vi "GUI_HTT_1Wire.vi"() -> ()   [LabVIEW 2013]
uses:
  Shared/GUI_Template/GUI_master/tcp_new_data_event.ctl
  Shared/GUI_Template/GUI_master/tcp new data cluster.ctl
panel:
  in  "Position.Channel 10::1":T1(ring) caption="Beamstop South"
  in  "Position.Channel 9::1":T1(ring) caption="Beamstop North"
  in  "Position.Channel 5::1":T1(ring) caption="Amp3 North"
  in  "Position.Channel 8::1":T1(ring) caption="Amp4 South"
  in  "Position.Channel 6::1":T1(ring) caption="Amp3 South"
  in  "Position.Channel 7::1":T1(ring) caption="Amp4 North"
  in  "Position.Channel 4::1":T1(ring) caption="Amp2 South"
  in  "Position.Channel 3::1":T1(ring) caption="Amp2 North"
  in  "Position.Channel 2::1":T1(ring) caption="Revo 1 South"
  in  "Position.Channel 1::1":T1(ring) caption="Revo 1 North"
  out "error IO 2":errorcluster
  out "tcp data event":T2
  in  "UDP error message":string
  in  "GUIdevice 2":string
  in  "GUIdevice 1":string="HTT-1Wire-LCave"
  in  "stop":bool
  # "HTT-1Wire"
  # "Energy"
  # "CAP"
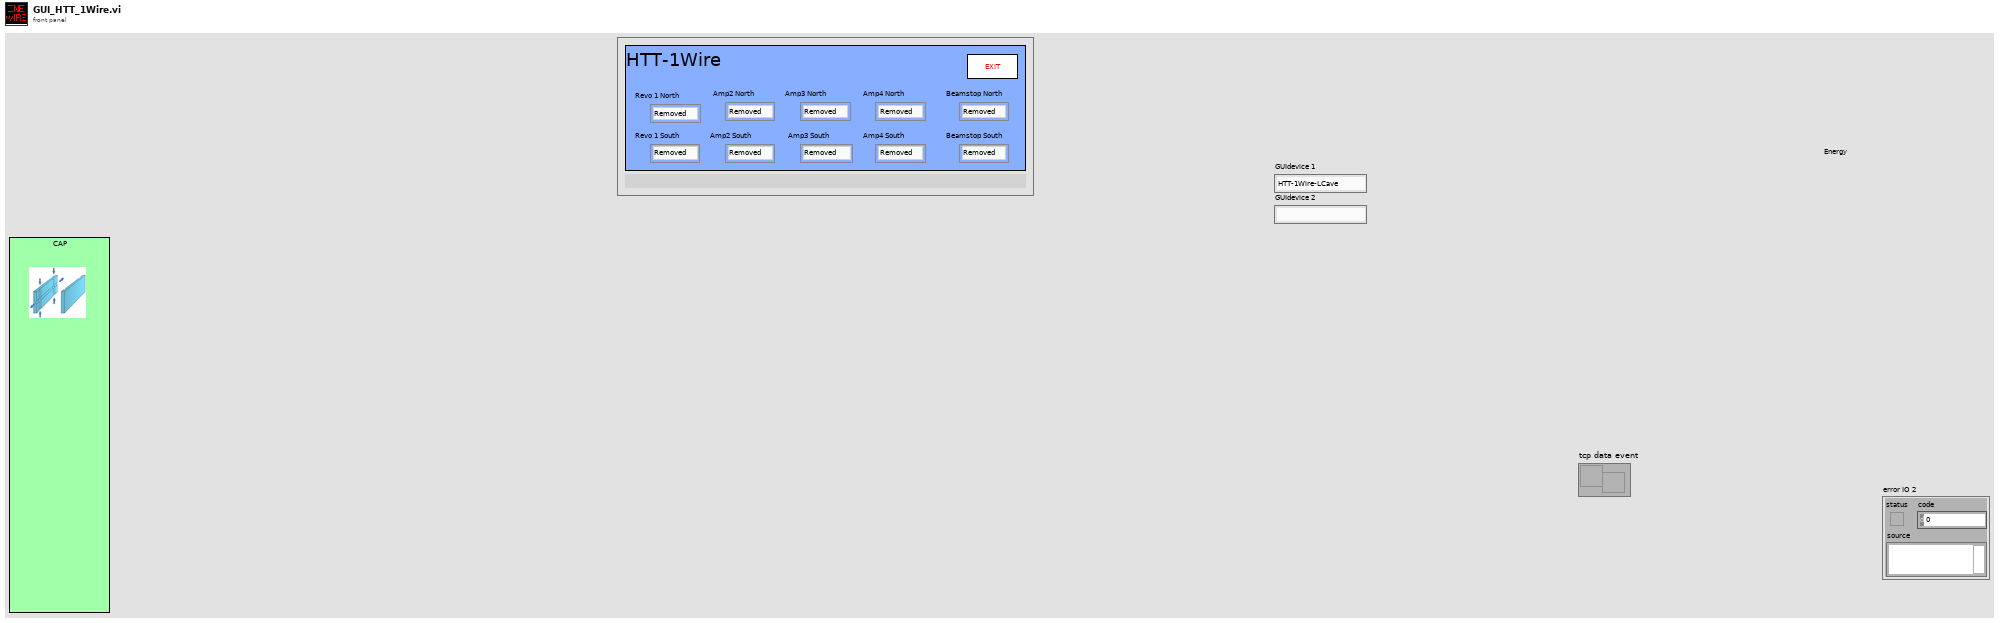
[diagram p1: front panel]
types:
  T1 = enum16{"Removed", "Inserted", "Unknown", "Moving"}
  T2 = typedef "tcp_new_data_event.ctl" = refnum<user-event>
  T3 = typedef "tcp new data cluster.ctl" = cluster{"EventEnum":enum16{"new data", "connection status update"}, "Device name":string}
  T4 = enum32{"invalid app kind", "Development System", "Run Time System", "Student Edition", "Embedded LabVIEW", "Evaluation", "Custom"}
  T5 = enum32{"Invalid", "Standard", "Closed", "Hidden", "Minimized", "Maximized"}
  T6 = cluster{"Core":cluster{"Current VI Reference":refnum<vi>, "Close Panel on Exit?":bool}, "Heater timing offset":dbl, "Discharge timing offset":dbl, "Jet trigger":bool, "Tik1":u32, "Tik2":u32, "Fire Continues Allowed":bool, "Jet enable":bool}
  T7 = cluster{"Current VI Reference":refnum<vi>, "Close Panel on Exit?":bool}
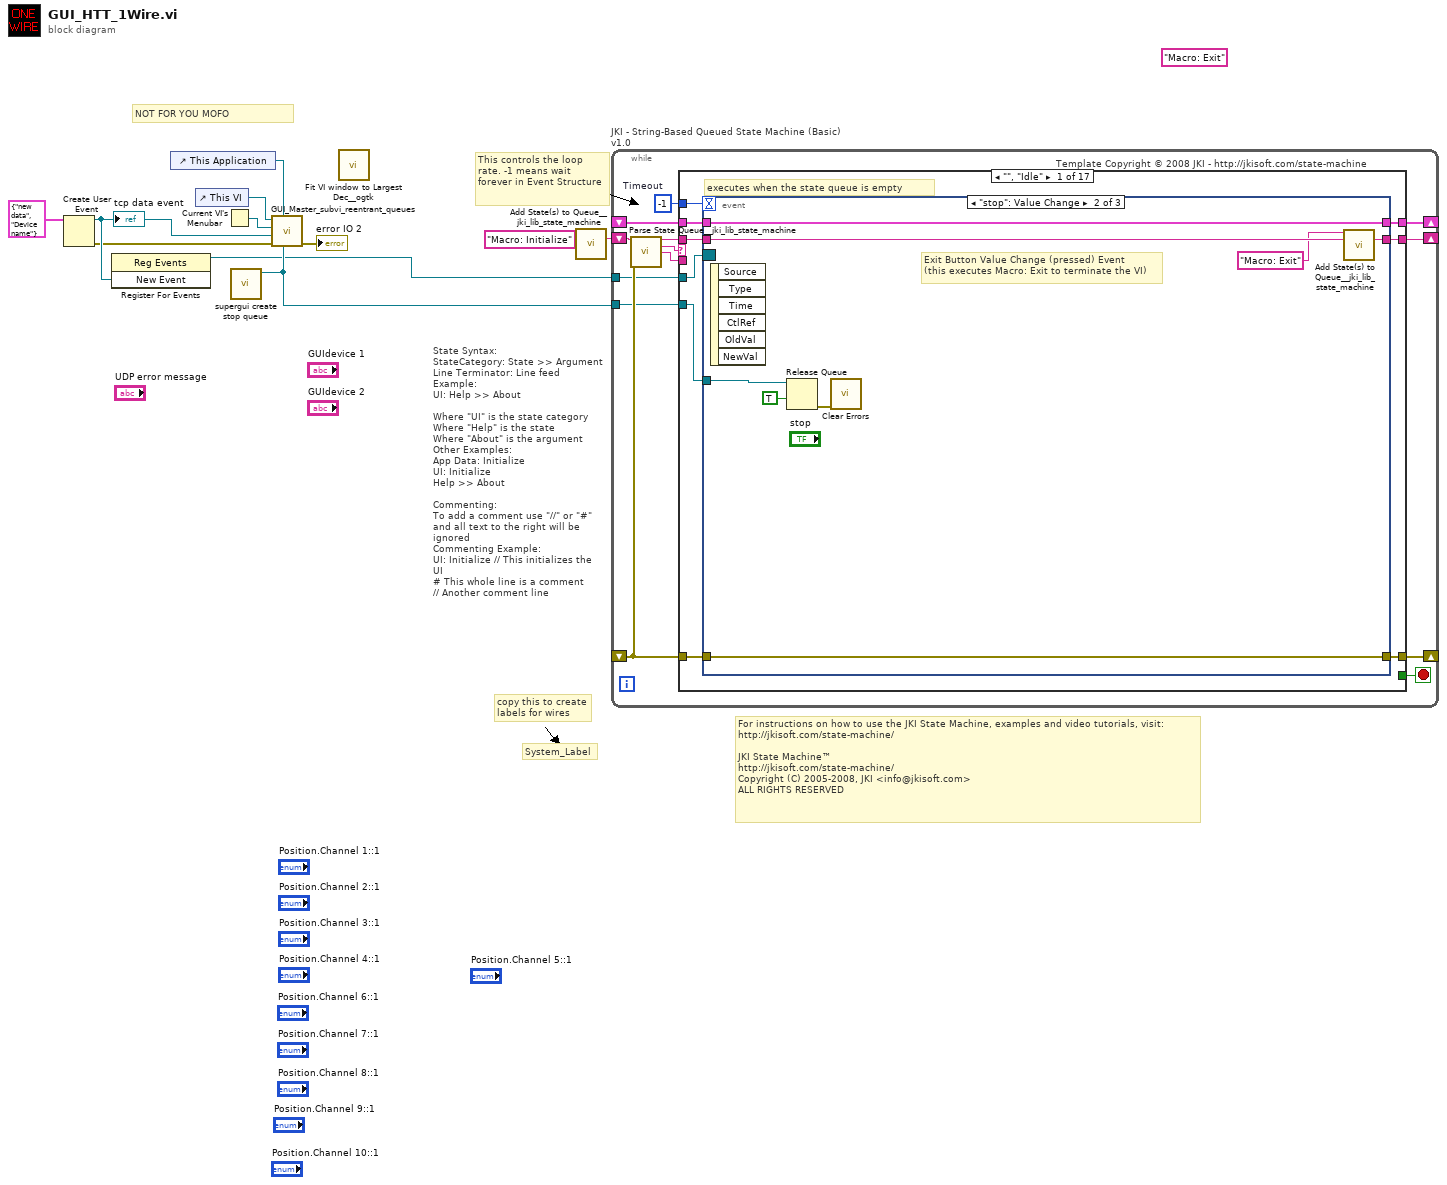
[diagram p0: block diagram]
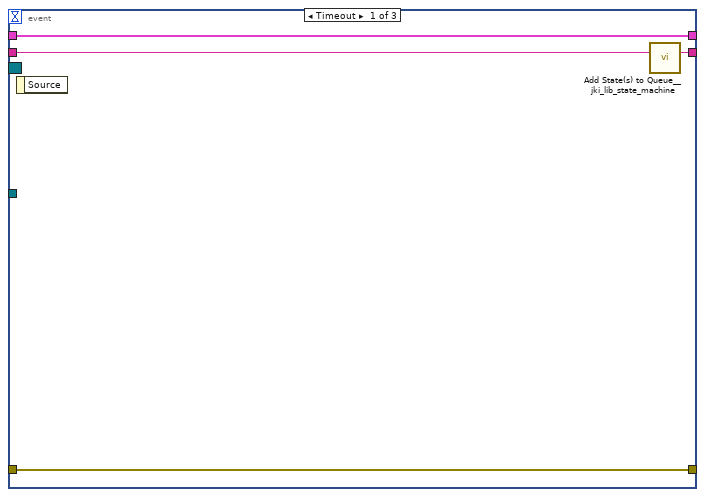
[diagram p2: hidden frame]
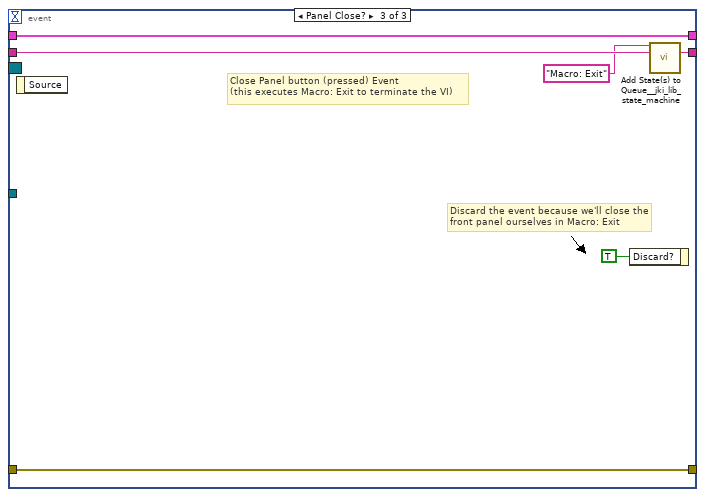
[diagram p3: hidden frame]
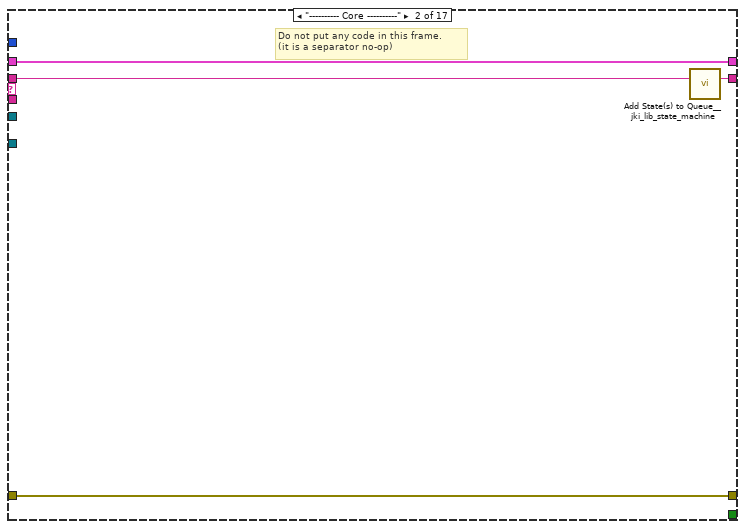
[diagram p4: hidden frame]
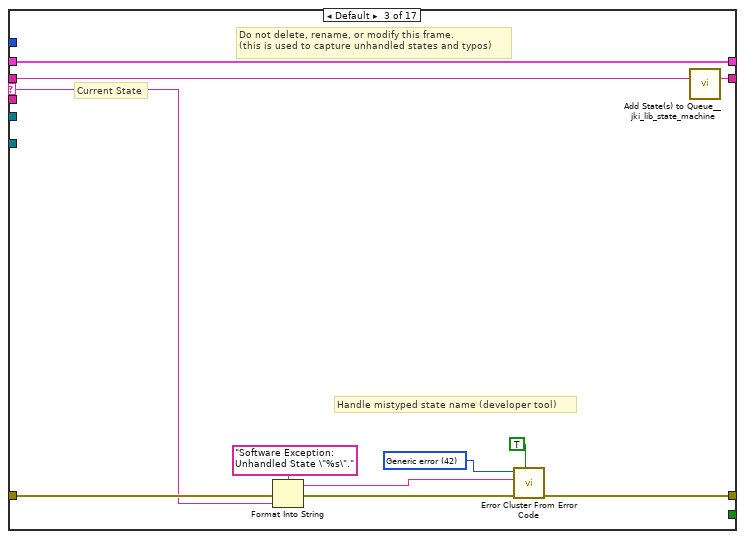
[diagram p5: hidden frame]
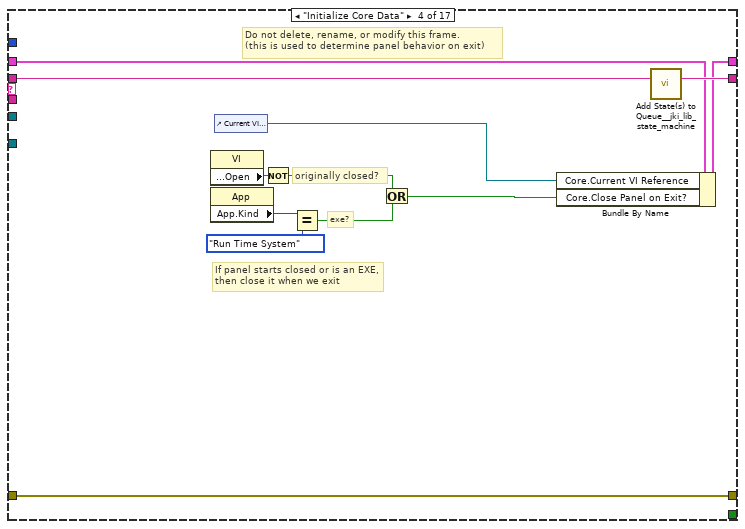
[diagram p6: hidden frame]
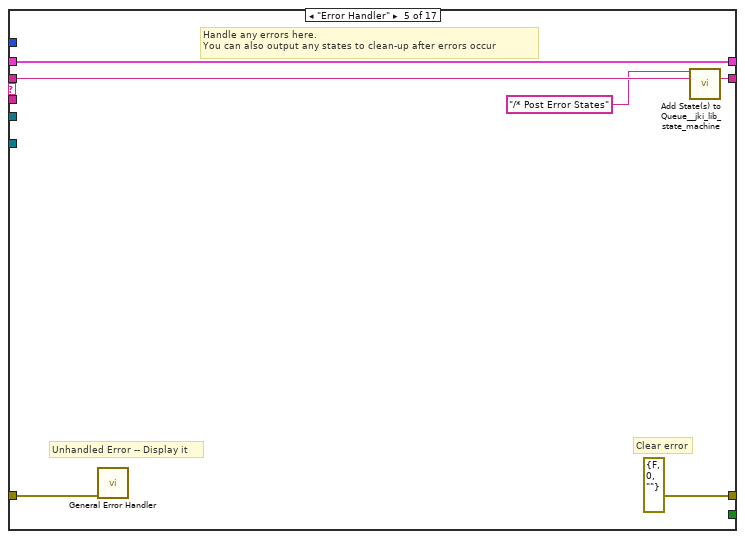
[diagram p7: hidden frame]
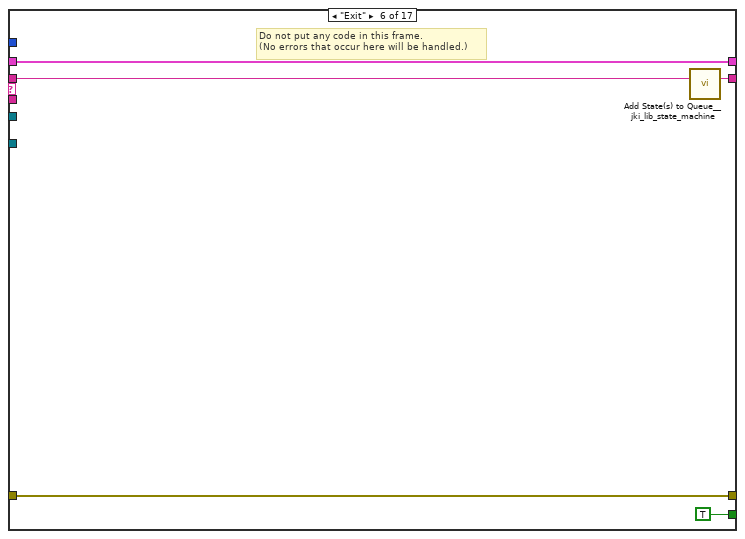
[diagram p8: hidden frame]
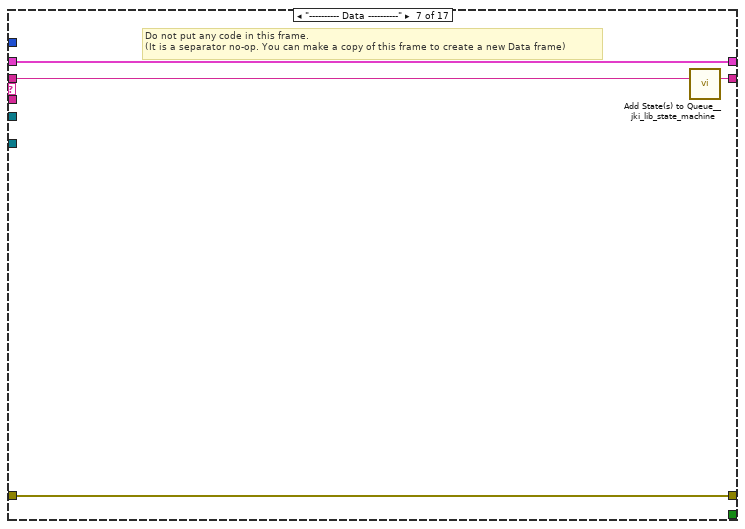
[diagram p9: hidden frame]
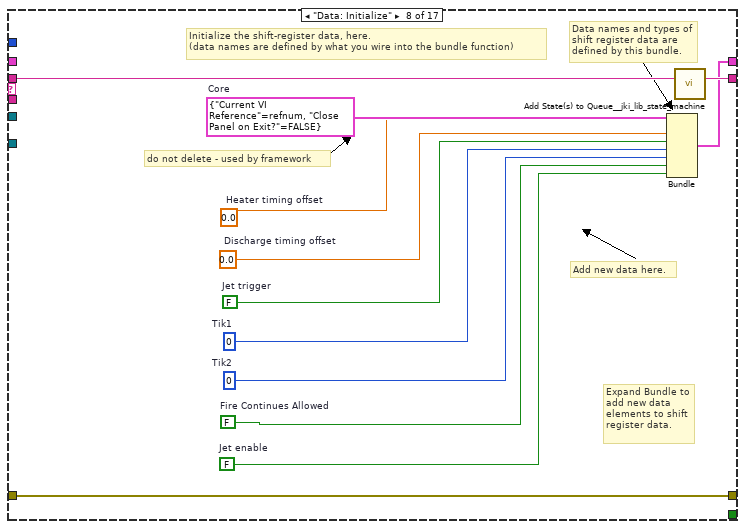
[diagram p10: hidden frame]
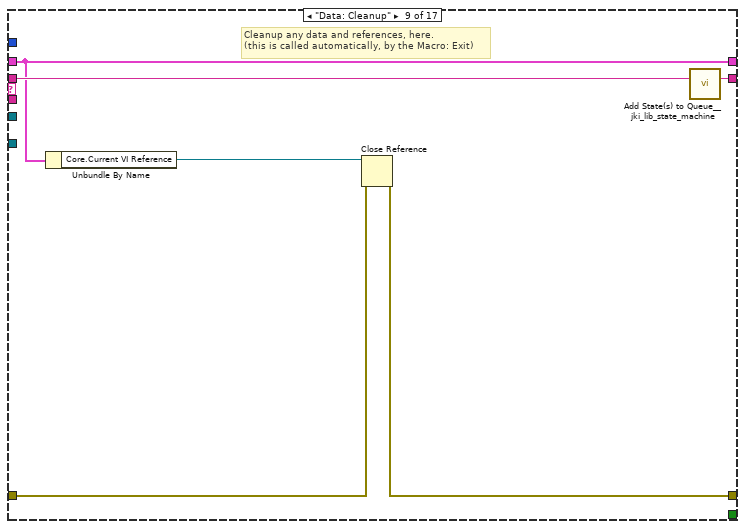
[diagram p11: hidden frame]
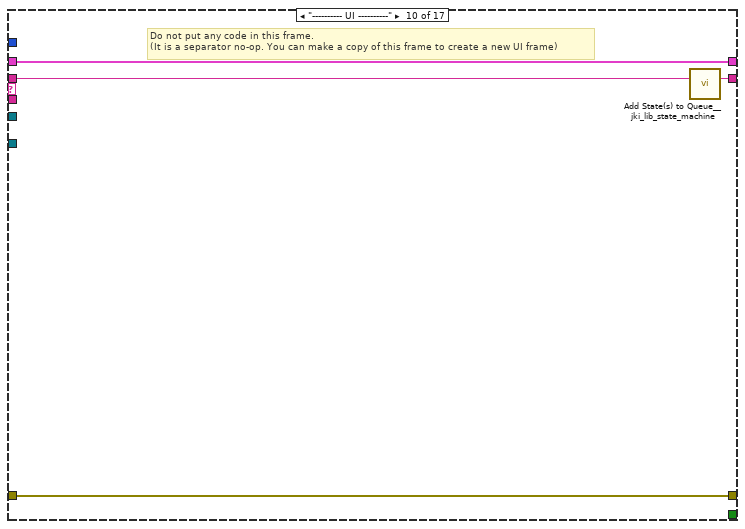
[diagram p12: hidden frame]
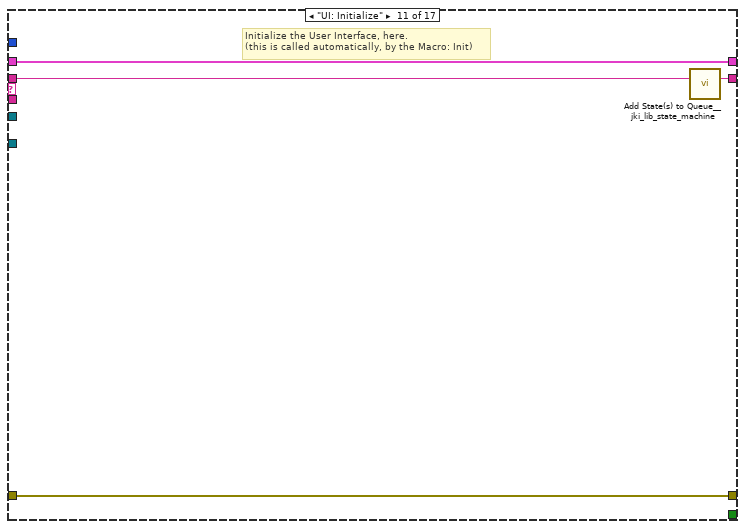
[diagram p13: hidden frame]
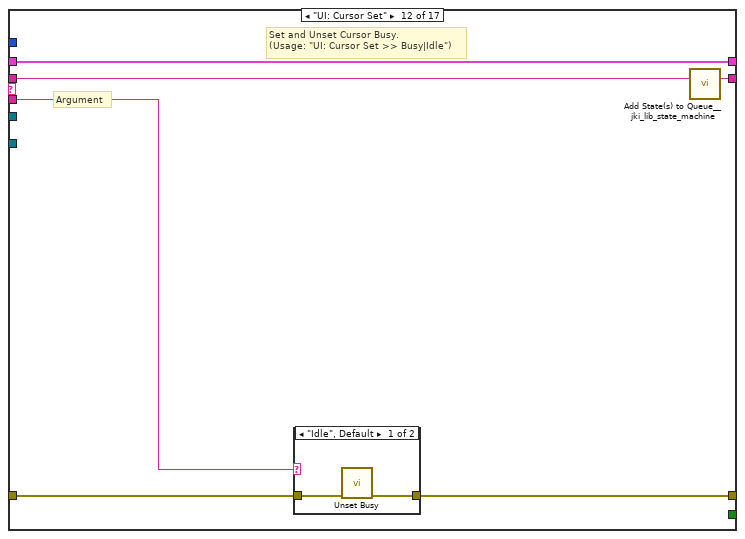
[diagram p14: hidden frame]
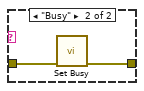
[diagram p15: hidden frame]
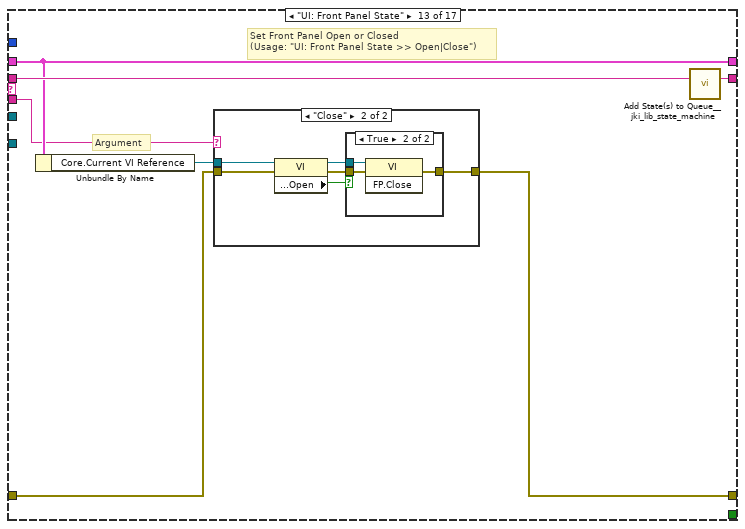
[diagram p16: hidden frame]
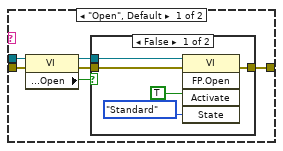
[diagram p17: hidden frame]
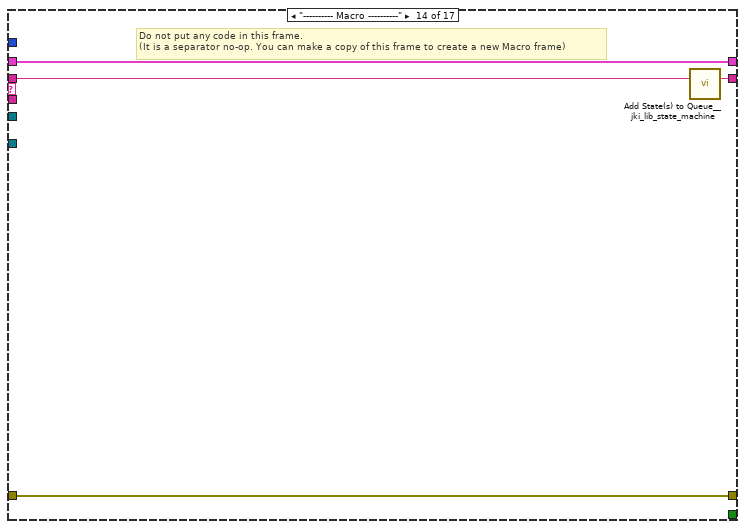
[diagram p20: hidden frame]
diagram:
  (unwired) "Macro: Exit"
  # "For instructions on how to use the JKI State Machine, examples and video tutorials, visit:\nhttp://jkisoft.com/state-machine/\n\nJKI State Machine™\nhttp://jkisoft.com/state-machine/\nCopyright (C) 2005-2008, JKI <info@jkisoft.com>\nALL RIGHTS RESERVED"
  # "State Syntax:\nStateCategory: State >> Argument\nLine Terminator: Line feed\nExample:\nUI: Help >> About\n\nWhere \"UI\" is the state category\nWhere \"Help\" is the state\nWhere \"About\" is the argument\nOther Examples:\nApp Data: Initialize\nUI: Initialize\nHelp >> About\n\nCommenting:\nTo add a comment use \"//\" or \"#\" and all text to the right will be ignored\nCommenting Example:\nUI: Initialize // This initializes the UI\n# This whole line is a comment\n// Another comment line"
  # "copy this to create labels for wires"
  # "This controls the loop rate. -1 means wait forever in Event Structure"
  # "System_Label"
  # "NOT FOR YOU MOFO"
  n1 = Create User Event(user event datatype=T3 {"EventEnum"=enum."new data", "Device name"="Device name"} ("New Event")) -> (user event=w10:refnum<user-event>, error out=w9:errorcluster)  [unwired: 1 in]
  "tcp data event" <- w10
  n2 = register-events(w10) -> (reference out=w1:refnum<event-registration>)  [unwired: 2 in, 1 out]
  n3 = control-ref of="This Application"() -> (w11:refnum<vi>)
  n4 = control-ref of="This VI"() -> (w5:refnum<vi>)
  n5 = Current VI's Menubar() -> (w7:refnum<k9>)
  n6 = call "supergui create stop queue.vi"() -> ("STOP Queue out"=w2:refnum<queue>)  [unwired: 11 in]
  n7 = call "GUI_Master_subvi_reentrant_queues.vi"("STOP Queue in"=w2, "This Application"=w11, "error in (no error)"=w9, "tcp data event"=w10, "Caller menu reference"=w7, "Caller VI ref"=w5) -> ("error out"=→"error IO 2":errorcluster)  [unwired: 5 in]
  n8 = call <userlib>:"Fit VI window to Largest Dec__ogtk.vi"() -> ()  [unwired: 6 in, 2 out]
  n9 = call <vilib>:"Add State(s) to Queue__jki_lib_state_machine.vi"("State(s) in (\"\")"="Macro: Initialize") -> ("States Out"=w3:string)  [unwired: 14 in]
  n10 = while "JKI - String-Based Queued State Machine (Basic) v1.0" {
    shift-right: [w17] -> _
    shift-left: _ -> [w16]
    shift-right: [w20] -> _
    shift-left: _ -> [w14]
    shift-right: [w19] -> _
    shift-left: w3 -> [w21]
    tunnel: w1 -> [w13]
    tunnel: w2 -> [w12]
    stop <- w18 stop-if-true
    w15 = -1  # Timeout
    # "Template Copyright © 2008 JKI - http://jkisoft.com/state-machine"
    n11 = call <vilib>:"Parse State Queue__jki_lib_state_machine.vi"("State Queue"=w21, "Error In (no error)"=w14) -> ("Remaining States"=w23:string, "Current State"=w24:string, "Arguments"=w22:string)  [unwired: 11 in]
    n12 = case shown="\"\", \"Idle\"" w24 {
      selector: w24 -> [_ _ w56 _ _ _ _ _ _ _ _ _ _ _ _ _ _]
      tunnel: w23 -> [w33 w55 w60 w78 w84 w89 w93 w105 w111 w115 w119 w125 w136 w162 w167 w177 w181]
      tunnel: w22 -> [_ _ _ _ _ _ _ _ _ _ _ w120 w130 _ _ _ _]
      tunnel: w16 -> [w31 w52 w58 w69 w81 w87 w90 _ w106 w112 w117 w123 w132 w159 w164 w174 w178]
      tunnel: [w30 w53 w62 w75 errorcluster {"status"=FALSE, "code"=0, "source"=""} ("error out") w86 w91 w102 w107 w113 w116 w121 w133 w160 w165 w175 w179] -> w20
      tunnel: w14 -> [w29 w53 w61 w75 w80 w86 w91 w102 w108 w113 w116 w122 w134 w160 w165 w175 w179]
      tunnel: [w32 w54 w59 w77 w83 w88 w92 w104 w110 w114 w118 w124 w135 w161 w166 w176 w180] -> w19
      tunnel: [_ _ _ _ _ TRUE _ _ _ _ _ _ _ _ _ _ _] -> w18
      tunnel: [w25 w52 w58 w76 w81 w87 w90 w103 w106 w112 w117 w123 w132 w159 w164 w174 w178] -> w17
      tunnel: w15 -> [w28 _ _ _ _ _ _ _ _ _ _ _ _ _ _ _ _]
      tunnel: w13 -> [w27 _ _ _ _ _ _ _ _ _ _ _ _ _ _ _ _]
      tunnel: w12 -> [w26 _ _ _ _ _ _ _ _ _ _ _ _ _ _ _ _]
      frame "", "Idle" {
        # "executes when the state queue is empty"
        n13 = event shown="[1] \"stop\": Value Change" {
          selector: w27 -> [_ _ _]
          dyn-events: _ -> [_ _ _]
          timeout: w28 -> [_ _ _]
          tunnel: w33 -> [w37 w45 w51]
          tunnel: [w36 w44 w50] -> w32
          tunnel: w31 -> [w34 w42 w48]
          tunnel: [w35 w43 w49] -> w30
          tunnel: w29 -> [w35 w43 w49]
          tunnel: [w34 w42 w48] -> w25
          tunnel: w26 -> [_ w39 _]
          event Timeout {
            n14 = event-data() -> ()  [unwired: 1 in, 1 out]
            n15 = call <vilib>:"Add State(s) to Queue__jki_lib_state_machine.vi"("State(s) in (\"\")"=w37) -> ("States Out"=w36:string)  [unwired: 14 in]
          }
          event "stop": Value Change {
            # "Exit Button Value Change (pressed) Event\n(this executes Macro: Exit to terminate the VI)"
            n16 = event-data() -> ()  [unwired: 1 in, 6 out]
            n17 = Release Queue(queue=w39, force destroy? (F)=TRUE) -> (error out=w40:errorcluster)  [unwired: 1 in, 2 out]
            n18 = call <vilib>:"Clear Errors.vi"("error in (no error)"=w40) -> ()  [unwired: 6 in, 1 out]
            n19 = call <vilib>:"Add State(s) to Queue__jki_lib_state_machine.vi"("State(s) in Front (\"\")"="Macro: Exit", "State(s) in (\"\")"=w45) -> ("States Out"=w44:string)  [unwired: 13 in]
          }
          event Panel Close? {
            # "Discard the event because we'll close the front panel ourselves in Macro: Exit"
            # "Close Panel button (pressed) Event\n(this executes Macro: Exit to terminate the VI)"
            n20 = event-data() -> ()  [unwired: 1 in, 1 out]
            n21 = event-data("Discard?"=TRUE) -> ()  [unwired: 1 in, 1 out]
            n22 = call <vilib>:"Add State(s) to Queue__jki_lib_state_machine.vi"("State(s) in Front (\"\")"="Macro: Exit", "State(s) in (\"\")"=w51) -> ("States Out"=w50:string)  [unwired: 13 in]
          }
        }
      }
      frame "---------- Core ----------" {
        # "Do not put any code in this frame.\n(it is a separator no-op)"
        n23 = call <vilib>:"Add State(s) to Queue__jki_lib_state_machine.vi"("State(s) in (\"\")"=w55) -> ("States Out"=w54:string)  [unwired: 14 in]
      }
      frame Default {
        w65 = 42 items=["No error", "Argument error", "Memory is full", "Out of zone", "End of file", "File already open", "Generic file I/O error", "File not found", "File permission error", "Disk is full", "Duplicate path", "Too many files open", "System feature not enabled", "Resource file not found", "Cannot add resource", "Resource not found", "Image not found", "Image memory error", "Pen does not exist", "Config type invalid", "Config token not found", "Config parse error", "Config memory error", "Bad external code format", "Bad external code offset", "External code not present", "Null window", "Destroy window error", "Null menu", "Print aborted", "Bad print record", "Print driver error", "Windows error during printing", "Memory error during printing", "Print dialog error", "Generic print error", "Invalid device refnum", "Device not found", "Device parameter error", "Device unit error", "Cannot open device", "Device call aborted", "Generic error", "Cancelled by user", "Object ID too low", "Object ID too high", "Object not in heap", "Unknown heap", "Unknown object (invalid DefProc)", "Unknown object (DefProc not in table)", "Message out of range", "Invalid (null) method", "Unknown message", "Manager call not supported", "Bad address", "Network operation in progress", "Network operation timed out", "Connection is busy", "Network attribute not supported", "Network error", "Address in use", "System out of memory", "Connection aborted", "Connection refused", "Not connected", "Already connected", "Connection closed", "Initialization error (interapplication manager)", "Bad occurrence", "Wait on unbound occurrence handler", "Occurrence queue overflow", "Datalog type conflict", "Unused", "Unrecognized type (interapplication manager)", "Memory corrupt", "Failed to make temporary DLL", "Old CIN version", "Drag socket not found", "Failed to load drop-object", "Failed to register OLE object", "Failed to release OLE object", "Format specifier type mismatch", "Unknown format specifier", "Too few format specifiers", "Too many format specifiers", "Scan failed", "Newer CIN version", "Error converting to variant", "Runtime menu error", "Password tampered", "Variant attribute not found", "Incompatible variant data type", "Event data is not available", "Event Store is not present", "Occurrence is not found", "Event Queue is not created", "Event info is not available", "Refnum passed is NULL", "Error retrieving Class GUID", "Error retrieving CoClass GUID", "Error retrieving TypeLib GUID.", "Bad built application magic bytes.", "Specific driver is different from the specific driver associated with the Logical Name.", "There is no session opened to the class driver.", "Max Error", "MAX - Error with config objects", "MAX - Error loading configuration", "MAX - Group not supported"]
        # "Current State"
        # "Do not delete, rename, or modify this frame.\n(this is used to capture unhandled states and typos)"
        # "Handle mistyped state name (developer tool)"
        n24 = Format Into String(format string="Software Exception: Unhandled State \"%s\"." ("message"), error in=w61, w56) -> (resulting string=w64:string, error out=w63:errorcluster)  [unwired: 1 in]
        n25 = call <vilib>:"Error Cluster From Error Code.vi"("show call chain? (False)"=TRUE, "error in (no error)"=w63, "error message (\"\")"=w64, "error code (0)"=w65) -> ("error out"=w62:errorcluster)  [unwired: 5 in]
        n26 = call <vilib>:"Add State(s) to Queue__jki_lib_state_machine.vi"("State(s) in (\"\")"=w60) -> ("States Out"=w59:string)  [unwired: 14 in]
      }
      frame "Initialize Core Data" {
        # "Do not delete, rename, or modify this frame.\n(this is used to determine panel behavior on exit)"
        # "originally closed?"
        # "exe?"
        # "If panel starts closed or is an EXE, then close it when we exit"
        n27 = property class="VI"() -> ("Front Panel.Open"=w74:bool)  [unwired: 2 in, 2 out]
        n28 = property class="App"() -> ("App.Kind"=w73:T4)  [unwired: 2 in, 2 out]
        n29 = control-ref of="Current VI Reference"() -> (w67:refnum<vi>)
        n30 = Not(x=w74) -> (.not. x?=w71:bool)
        n31 = Equal?(x=w73, y=T4."Run Time System" ("Application:Kind")) -> (x = y?=w70:bool)
        n32 = Or(x=w71, y=w70) -> (x .or. y?=w68:bool)
        n33 = Bundle By Name(cluster=w69, "Core.Current VI Reference"=w67, "Core.Close Panel on Exit?"=w68) -> (w76:T6)
        n34 = call <vilib>:"Add State(s) to Queue__jki_lib_state_machine.vi"("State(s) in (\"\")"=w78) -> ("States Out"=w77:string)  [unwired: 14 in]
      }
      frame "Error Handler" {
        # "Unhandled Error -- Display it"
        # "Handle any errors here.\nYou can also output any states to clean-up after errors occur"
        # "Clear error"
        n35 = call <vilib>:"General Error Handler.vi"("error in (no error)"=w80) -> ()  [unwired: 10 in, 5 out]
        n36 = call <vilib>:"Add State(s) to Queue__jki_lib_state_machine.vi"("State(s) in Front (\"\")"="/* Post Error States", "State(s) in (\"\")"=w84) -> ("States Out"=w83:string)  [unwired: 13 in]
      }
      frame "Exit" {
        # "Do not put any code in this frame.\n(No errors that occur here will be handled.)"
        n37 = call <vilib>:"Add State(s) to Queue__jki_lib_state_machine.vi"("State(s) in (\"\")"=w89) -> ("States Out"=w88:string)  [unwired: 14 in]
      }
      frame "---------- Data ----------" {
        # "Do not put any code in this frame.\n(It is a separator no-op. You can make a copy of this frame to create a new Data frame)"
        n38 = call <vilib>:"Add State(s) to Queue__jki_lib_state_machine.vi"("State(s) in (\"\")"=w93) -> ("States Out"=w92:string)  [unwired: 14 in]
      }
      frame "Data: Initialize" {
        w94 = FALSE  # Jet enable
        w95 = FALSE  # Fire Continues Allowed
        w97 = u32 0  # Tik1
        w96 = u32 0  # Tik2
        w98 = FALSE  # Jet trigger
        w99 = 0.0  # Discharge timing offset
        w100 = 0.0  # Heater timing offset
        w101 = T7 {"Current VI Reference"=refnum, "Close Panel on Exit?"=FALSE}  # Core
        # "do not delete - used by framework"
        # "Expand Bundle to add new data elements to shift register data."
        # "Add new data here."
        # "Data names and types of shift register data are defined by this bundle."
        # "Initialize the shift-register data, here.\n(data names are defined by what you wire into the bundle function)"
        n39 = Bundle("Core"=w101, "Heater timing offset"=w100, "Discharge timing offset"=w99, "Jet trigger"=w98, "Tik1"=w97, "Tik2"=w96, "Fire Continues Allowed"=w95, "Jet enable"=w94) -> (w103:T6)  [unwired: 1 in]
        n40 = call <vilib>:"Add State(s) to Queue__jki_lib_state_machine.vi"("State(s) in (\"\")"=w105) -> ("States Out"=w104:string)  [unwired: 14 in]
      }
      frame "Data: Cleanup" {
        # "Cleanup any data and references, here.\n(this is called automatically, by the Macro: Exit)"
        n41 = Unbundle By Name(w106) -> ("Core.Current VI Reference"=w109:refnum<vi>)
        n42 = Close Reference(reference=w109, error in (no error)=w108) -> (error out=w107:errorcluster)
        n43 = call <vilib>:"Add State(s) to Queue__jki_lib_state_machine.vi"("State(s) in (\"\")"=w111) -> ("States Out"=w110:string)  [unwired: 14 in]
      }
      frame "---------- UI ----------" {
        # "Do not put any code in this frame.\n(It is a separator no-op. You can make a copy of this frame to create a new UI frame)"
        n44 = call <vilib>:"Add State(s) to Queue__jki_lib_state_machine.vi"("State(s) in (\"\")"=w115) -> ("States Out"=w114:string)  [unwired: 14 in]
      }
      frame "UI: Initialize" {
        # "Initialize the User Interface, here.\n(this is called automatically, by the Macro: Init)"
        n45 = call <vilib>:"Add State(s) to Queue__jki_lib_state_machine.vi"("State(s) in (\"\")"=w119) -> ("States Out"=w118:string)  [unwired: 14 in]
      }
      frame "UI: Cursor Set" {
        # "Argument"
        # "Set and Unset Cursor Busy.\n(Usage: \"UI: Cursor Set >> Busy|Idle\")"
        n46 = case shown="\"Idle\", Default" w120 {
          tunnel: w122 -> [w127 w129]
          tunnel: [w126 w128] -> w121
          frame "Idle", Default {
            n47 = call <vilib>:"Unset Busy.vi"("error in (no error)"=w127) -> ("error out"=w126:errorcluster)  [unwired: 10 in]
          }
          frame "Busy" {
            n48 = call <vilib>:"Set Busy.vi"("error in (no error)"=w129) -> ("error out"=w128:errorcluster)  [unwired: 9 in, 1 out]
          }
        }
        n49 = call <vilib>:"Add State(s) to Queue__jki_lib_state_machine.vi"("State(s) in (\"\")"=w125) -> ("States Out"=w124:string)  [unwired: 14 in]
      }
      frame "UI: Front Panel State" {
        # "Argument"
        # "Set Front Panel Open or Closed\n(Usage: \"UI: Front Panel State >> Open|Close\")"
        n50 = Unbundle By Name(w132) -> ("Core.Current VI Reference"=w131:refnum<vi>)
        n51 = case shown="\"Close\"" w130 {
          tunnel: w134 -> [w140 w153]
          tunnel: [w142 w154] -> w133
          tunnel: w131 -> [w141 w151]
          frame "Open", Default {
            n52 = property class="VI"(reference=w141, error in=w140) -> (reference out=w138:refnum<vi>, error out=w139:errorcluster, "Front Panel.Open"=w137:bool)
            n53 = case shown="False" w137 {
              tunnel: [w145 w148] -> w142
              tunnel: w139 -> [w144 w148]
              tunnel: w138 -> [w143 _]
              frame False {
                n54 = invoke class="VI" method="FP.Open"(reference=w143, error in=w144, "Activate"=TRUE, "State"=T5."Standard") -> (error out=w145:errorcluster)  [unwired: 1 in, 4 out]
              }
              frame True {
              }
            }
          }
          frame "Close" {
            n55 = property class="VI"(reference=w151, error in=w153) -> (reference out=w150:refnum<vi>, error out=w152:errorcluster, "Front Panel.Open"=w149:bool)
            n56 = case shown="True" w149 {
              tunnel: [w155 w158] -> w154
              tunnel: w152 -> [w155 w157]
              tunnel: w150 -> [_ w156]
              frame False {
              }
              frame True {
                n57 = invoke class="VI" method="FP.Close"(reference=w156, error in=w157) -> (error out=w158:errorcluster)  [unwired: 1 in, 2 out]
              }
            }
          }
        }
        n58 = call <vilib>:"Add State(s) to Queue__jki_lib_state_machine.vi"("State(s) in (\"\")"=w136) -> ("States Out"=w135:string)  [unwired: 14 in]
      }
      frame "---------- Macro ----------" {
        # "Do not put any code in this frame.\n(It is a separator no-op. You can make a copy of this frame to create a new Macro frame)"
        n59 = call <vilib>:"Add State(s) to Queue__jki_lib_state_machine.vi"("State(s) in (\"\")"=w162) -> ("States Out"=w161:string)  [unwired: 14 in]
      }
      frame "Macro: Initialize" {
        w163 = "Data: Initialize\nInitialize Core Data\nUI: Initialize\nUI: Front Panel State >> Open"  # Data: Initialize Initialize Core Data UI: Initialize UI: Front Panel State >> Open
        # "Initialization Macro\n(This is called once, when the VI starts)"
        n60 = call <vilib>:"Add State(s) to Queue__jki_lib_state_machine.vi"("State(s) in Front (\"\")"=w163, "State(s) in (\"\")"=w167) -> ("States Out"=w166:string)  [unwired: 13 in]
      }
      frame "Macro: Exit" {
        # "Exit Macro\n(This is called once, when the VI exits)"
        n61 = Unbundle By Name(w174) -> ("Core.Close Panel on Exit?"=w173:bool)
        n62 = Select(t="UI: Front Panel State >> Close", s=w173, f="") -> (s? t:f=w170:string)
        n63 = call <vilib>:"Add State(s) to Queue__jki_lib_state_machine.vi"("State(s) in (\"\")"=w170, "State(s) at Back (\"\")"="Data: Cleanup\nExit") -> ("States Out"=w168:string)  [unwired: 13 in]
        n64 = call <vilib>:"Add State(s) to Queue__jki_lib_state_machine.vi"("State(s) in Front (\"\")"=w168, "State(s) in (\"\")"=w177) -> ("States Out"=w176:string)  [unwired: 13 in]
      }
      frame "---------- New Category ----------" {
        # "Template Separator\n(You can make a copy of, or modify, this frame)"
        n65 = call <vilib>:"Add State(s) to Queue__jki_lib_state_machine.vi"("State(s) in (\"\")"=w181) -> ("States Out"=w180:string)  [unwired: 14 in]
      }
    }
  }
